vi "MoverMotoresFinalJoyStickDecorado.vi"() -> ()   [LabVIEW 2016]
uses:
  <vilib>/Instr/_visa.llb/VISA Configure Serial Port (Instr).vi
  <vilib>/Utility/inputDevices.llb/closeJoystick.vi
  <vilib>/Utility/inputDevices.llb/joystickAcquire.vi
panel:
  in  "Motor A":i64(knob) scale=-90.0..90.0
  out "XY Graph":cluster{"Y":dbl[], "Y":dbl[]}[](graph)
  in  "VISA resource name":refnum<visa-resource-name>
  out "z":dbl
  out "y":dbl
  out "x":dbl
  in  "L3":dbl
  in  "L2":dbl
  in  "L1":dbl
  in  "L0":dbl
  in  "Velocidad":u64(slide) scale=1.0..10.0
  out "Resultado":string caption="Result"
  in  "Motor C":i64(knob) scale=-90.0..90.0
  in  "Motor B":i64(knob) scale=-90.0..90.0
  in  "stop":bool
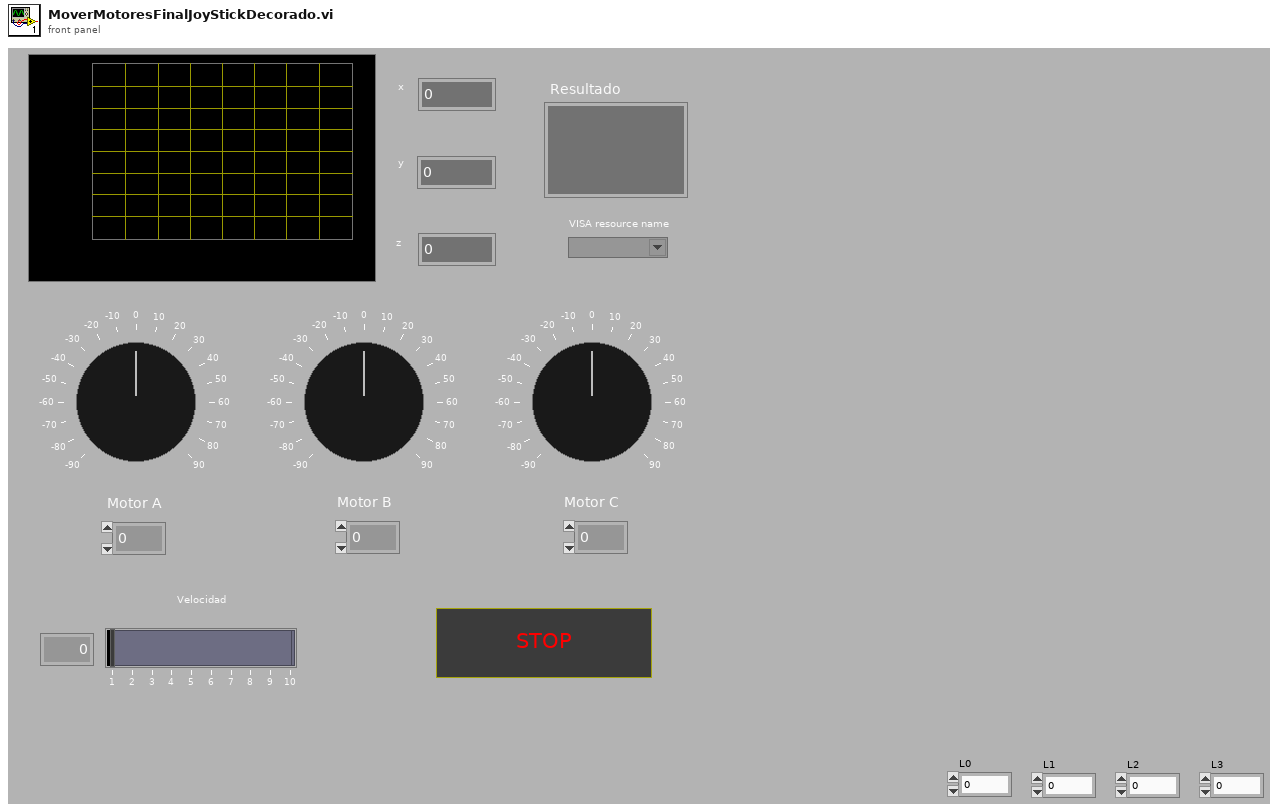
[diagram p1: front panel]
types:
  T1 = cluster{"button 1":bool, "button 2":bool, "button 3":bool, "button 4":bool, "button 5":bool, "button 6":bool, "button 7":bool, "button 8":bool, "button 9":bool, "button 10":bool, "button 11":bool, "button 12":bool, "button 13":bool, "button 14":bool, "button 15":bool, "button 16":bool, "button 17":bool, "button 18":bool, "button 19":bool, "button 20":bool, "button 21":bool, "button 22":bool, "button 23":bool, "button 24":bool, "button 25":bool, "button 26":bool, "button 27":bool, "button 28":bool, "button 29":bool, "button 30":bool, "button 31":bool, "button 32":bool}
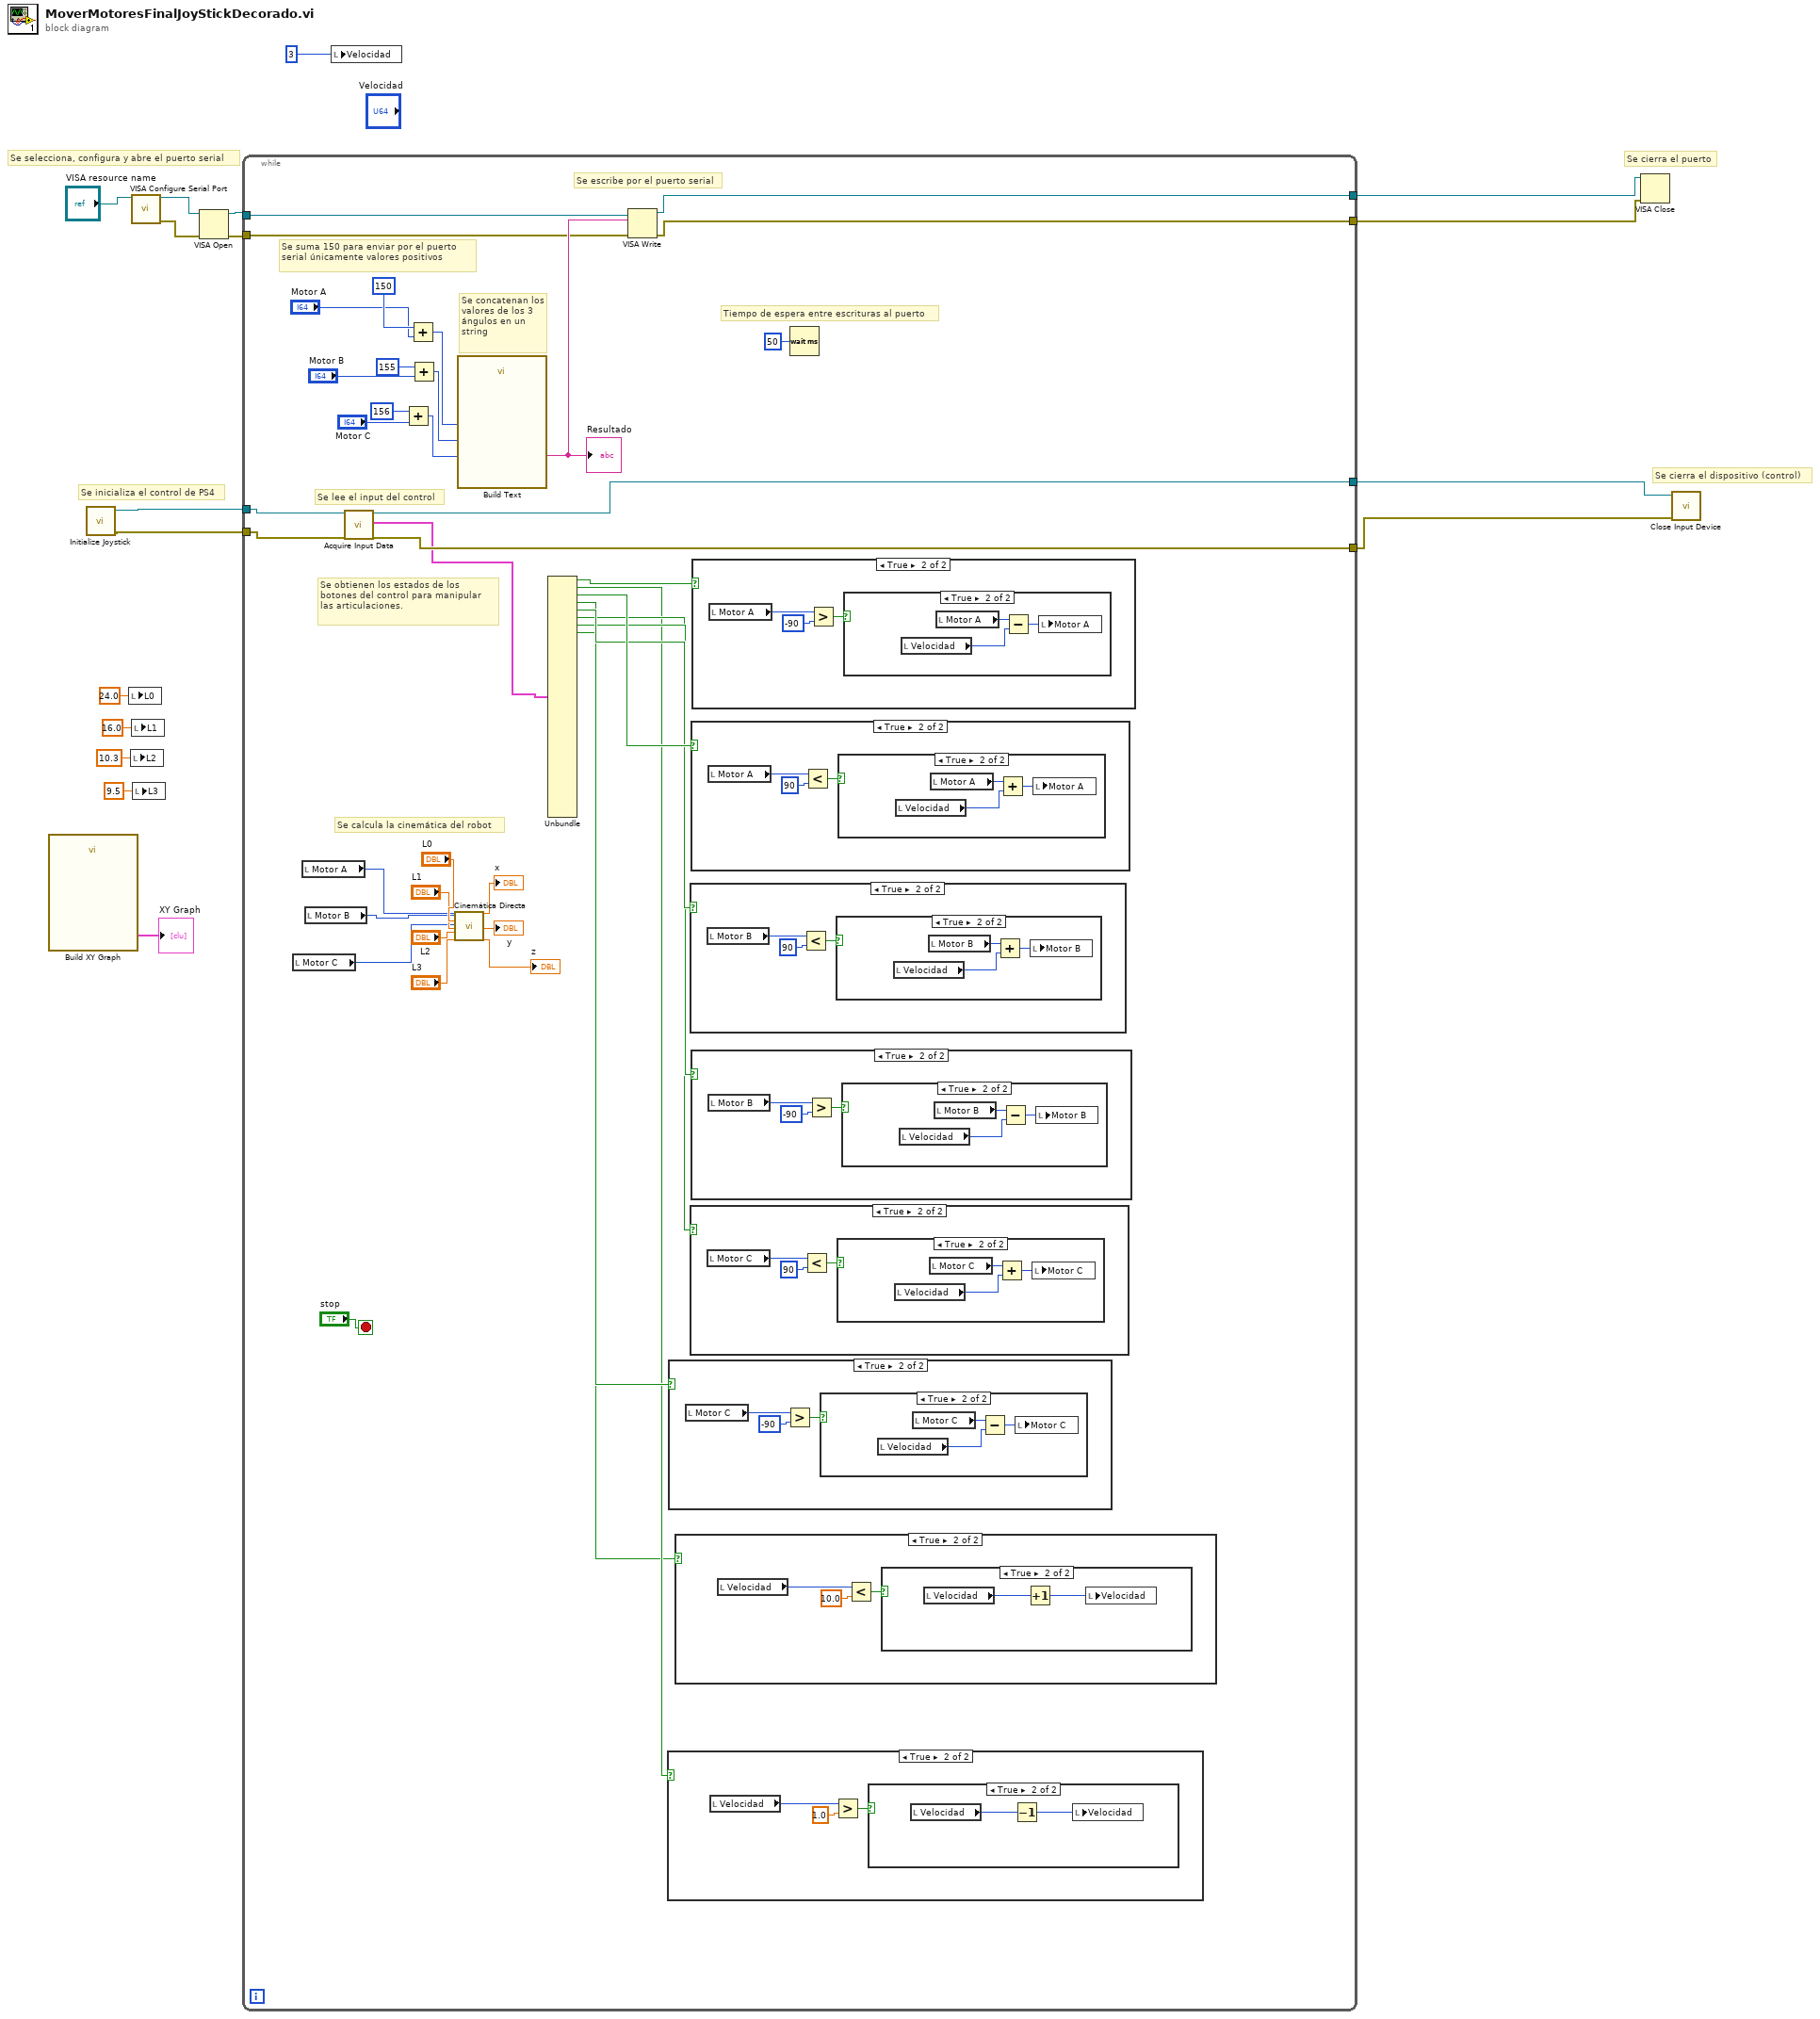
[diagram p0: block diagram]
diagram:
  # "Se cierra el dispositivo (control)"
  # "Se cierra el puerto"
  # "Se inicializa el control de PS4"
  # "Se selecciona, configura y abre el puerto serial"
  n1 = call "Build XY Graph"() -> ("XY Graph"=→"XY Graph":cluster{"X":dbl[], "Y":dbl[]}[])  [unwired: 10 in, 1 out]
  n2 = call <vilib>:"Initialize Joystick.vi"() -> ("error out"=w7:errorcluster, "device ID"=w8:refnum<k1>)  [unwired: 10 in]
  n3 = local write "L0"(24.0 ("L0")) -> ()
  n4 = local write "L2"(10.3 ("L2")) -> ()
  n5 = call-poly "VISA Configure Serial Port"("VISA resource name"="VISA resource name") -> ("VISA resource name out"=w15:refnum<visa-resource-name>, "error out"=w14:errorcluster)  [unwired: 13 in]
  n6 = local write "L1"(16.0 ("L1")) -> ()
  n7 = local write "L3"(9.5 ("L3")) -> ()
  n8 = VISA Open(error in (no error)=w14, VISA resource name=w15) -> (VISA resource name=w13:refnum<visa-resource-name>, error out=w12:errorcluster)  [unwired: 3 in]
  n9 = while {
    tunnel: w8 -> [w47]
    tunnel: w7 -> [w46]
    tunnel: [w45] -> w17
    tunnel: [w44] -> w5
    tunnel: w13 -> [w36]
    tunnel: w12 -> [w34]
    tunnel: [w33] -> w11
    tunnel: [w32] -> w10
    stop <- "stop" stop-if-true
    # "Se obtienen los estados de los botones del control para manipular las articulaciones."
    # "Tiempo de espera entre escrituras al puerto"
    # "Se lee el input del control"
    # "Se escribe por el puerto serial"
    # "Se concatenan los valores de los 3 ángulos en un string"
    # "Se suma 150 para enviar por el puerto serial únicamente valores positivos"
    # "Se calcula la cinemática del robot"
    n10 = local read "Motor C"() -> (w37:i64)
    n11 = local read "Motor A"() -> (w39:i64)
    n12 = local read "Motor B"() -> (w38:i64)
    n13 = call-poly <vilib>:"Acquire Input Data.vi"("device ID"=w47, "error in (no error)"=w46) -> ("device ID"=w45:refnum<k1>, "button info"=w23:T1, "error out"=w44:errorcluster)  [unwired: 13 in, 2 out]
    n14 = Add(x=i64 156, y="Motor C") -> (x+y=w49:i64)
    n15 = Add(x=150, y="Motor A") -> (x+y=w53:i64)
    n16 = Add(x=i64 155, y="Motor B") -> (x+y=w51:i64)
    n17 = call "Cinemática Directa.vi"("t1"=w39, "t2"=w38, "L0"="L0", "t3"=w37, "L1"="L1", "L2"="L2", "L3"="L3") -> ("x"=→"x":dbl, "y"=→"y":dbl, "z"=→"z":dbl)  [unwired: 18 in]
    n18 = call "Build Text"("motor1"=w53, "motor2"=w51, "motor3"=w49) -> ("Result"=w35:string)  [unwired: 11 in, 1 out]
    "Resultado" <- w35
    n19 = Unbundle(w23) -> ("button 1"=w31:bool, "button 2"=w25:bool, "button 3"=w30:bool, "button 4"=w24:bool, "button 5"=w29:bool, "button 6"=w27:bool, "button 7"=w28:bool, "button 8"=w26:bool)  [unwired: 24 out]
    n20 = VISA Write(VISA resource name=w36, write buffer=w35, error in (no error)=w34) -> (VISA resource name out=w33:refnum<visa-resource-name>, error out=w32:errorcluster)  [unwired: 1 out]
    n21 = case shown="True" w25 {
      frame False {
      }
      frame True {
        n22 = local read "Velocidad"() -> (w59:u64)
        n23 = Greater?(x=w59, y=1.0) -> (0:w58:bool)
        n24 = case shown="True" w58 {
          frame False {
          }
          frame True {
            n25 = local read "Velocidad"() -> (w61:u64)
            n26 = Decrement(x=w61) -> (x-1=w60:u64)
            n27 = local write "Velocidad"(w60) -> ()
          }
        }
      }
    }
    n28 = case shown="True" w26 {
      frame False {
      }
      frame True {
        n29 = local read "Motor C"() -> (w68:i64)
        n30 = Greater?(x=w68, y=i64 -90) -> (0:w69:bool)
        n31 = case shown="True" w69 {
          frame False {
          }
          frame True {
            n32 = local read "Velocidad"() -> (w71:u64)
            n33 = local read "Motor C"() -> (w72:i64)
            n34 = Subtract(x=w72, y=w71) -> (x-y=w70:u64)
            n35 = local write "Motor C"(w70) -> ()
          }
        }
      }
    }
    n36 = case shown="True" w24 {
      frame False {
      }
      frame True {
        n37 = local read "Velocidad"() -> (w64:u64)
        n38 = Less?(x=w64, y=10.0) -> (x < y?=w63:bool)
        n39 = case shown="True" w63 {
          frame False {
          }
          frame True {
            n40 = local read "Velocidad"() -> (w66:u64)
            n41 = Increment(x=w66) -> (x+1=w65:u64)
            n42 = local write "Velocidad"(w65) -> ()
          }
        }
      }
    }
    n43 = case shown="True" w29 {
      frame False {
      }
      frame True {
        n44 = local read "Motor B"() -> (w86:i64)
        n45 = Less?(x=w86, y=i64 90) -> (x < y?=w87:bool)
        n46 = case shown="True" w87 {
          frame False {
          }
          frame True {
            n47 = local read "Velocidad"() -> (w88:u64)
            n48 = local read "Motor B"() -> (w90:i64)
            n49 = Add(x=w90, y=w88) -> (x+y=w89:u64)
            n50 = local write "Motor B"(w89) -> ()
          }
        }
      }
    }
    n51 = case shown="True" w27 {
      frame False {
      }
      frame True {
        n52 = local read "Motor C"() -> (w74:i64)
        n53 = Less?(x=w74, y=i64 90) -> (x < y?=w75:bool)
        n54 = case shown="True" w75 {
          frame False {
          }
          frame True {
            n55 = local read "Velocidad"() -> (w77:u64)
            n56 = local read "Motor C"() -> (w78:i64)
            n57 = Add(x=w78, y=w77) -> (x+y=w76:u64)
            n58 = local write "Motor C"(w76) -> ()
          }
        }
      }
    }
    n59 = case shown="True" w30 {
      frame False {
      }
      frame True {
        n60 = local read "Motor A"() -> (w97:i64)
        n61 = Less?(x=w97, y=i64 90) -> (x < y?=w99:bool)
        n62 = case shown="True" w99 {
          frame False {
          }
          frame True {
            n63 = local read "Velocidad"() -> (w100:u64)
            n64 = local read "Motor A"() -> (w102:i64)
            n65 = Add(x=w102, y=w100) -> (x+y=w101:u64)
            n66 = local write "Motor A"(w101) -> ()
          }
        }
      }
    }
    n67 = case shown="True" w28 {
      frame False {
      }
      frame True {
        n68 = local read "Motor B"() -> (w80:i64)
        n69 = Greater?(x=w80, y=i64 -90) -> (0:w81:bool)
        n70 = case shown="True" w81 {
          frame False {
          }
          frame True {
            n71 = local read "Velocidad"() -> (w82:u64)
            n72 = local read "Motor B"() -> (w84:i64)
            n73 = Subtract(x=w84, y=w82) -> (x-y=w83:u64)
            n74 = local write "Motor B"(w83) -> ()
          }
        }
      }
    }
    n75 = case shown="True" w31 {
      frame False {
      }
      frame True {
        n76 = local read "Motor A"() -> (w92:i64)
        n77 = Greater?(x=w92, y=i64 -90) -> (0:w93:bool)
        n78 = case shown="True" w93 {
          frame False {
          }
          frame True {
            n79 = local read "Velocidad"() -> (w94:u64)
            n80 = local read "Motor A"() -> (w96:i64)
            n81 = Subtract(x=w96, y=w94) -> (x-y=w95:u64)
            n82 = local write "Motor A"(w95) -> ()
          }
        }
      }
    }
    n83 = Wait (ms)(milliseconds to wait=u32 50) -> ()  [unwired: 1 out]
  }
  n84 = local write "Velocidad"(u64 3 ("Velocidad\nVelocidad")) -> ()
  n85 = VISA Close(VISA resource name=w11, error in (no error)=w10) -> ()  [unwired: 1 out]
  n86 = call-poly <vilib>:"Close Input Device.vi"("error in (no error)"=w5, "device ID"=w17) -> ()  [unwired: 8 in, 1 out]
